vi "Test HighFrequency Client Connection.vi"() -> ()   [LabVIEW 2013]
uses:
  <vilib>/LabVIEW Open Source Project/MQTT Control Packets/Control Packets/CONNACK/Connect Return Code -- enum.ctl
  Server/Server class/Server.lvclass/Server.ctl
  Client/Client Class/Client.lvclass/Client.ctl
  <vilib>/LabVIEW Open Source Project/MQTT Control Packets/Control Packets/PUBLISH/PUBLISH.lvclass
  Server/Server class/Server.lvclass
  MQTT_Base/Base Class/MQTT_Base.lvclass
  Client/Client Class/Client.lvclass
  MQTT_TCP/Connection/TCPConnection.lvclass
  <vilib>/LabVIEW Open Source Project/MQTT Control Packets/Control Packets/CONNACK/CONNACK.lvclass
panel:
  out "NO RESPONSE":bool
  out "timed out?":bool
  out "Stop":dbl format="%.06f"
  out "Connect":dbl format="%.06f"
  out "Start":dbl format="%.06f"
  out "STOPPING":bool
  out "Waveform Chart":T1(graph)
  out "Loop period (s)":dbl format="%.06f"
  out "client Outgoing ID Request":i32
  out "Process Response":i32
  out "Process Incoming ID Request":i32
  out "Process Status":T2=enum."Server Unavailable"
  out "error server":errorcluster
  out "Client Status":T2=enum."Server Unavailable"
  out "error client process":errorcluster
  out "NbConnections":u32
  out "error client consumer":errorcluster
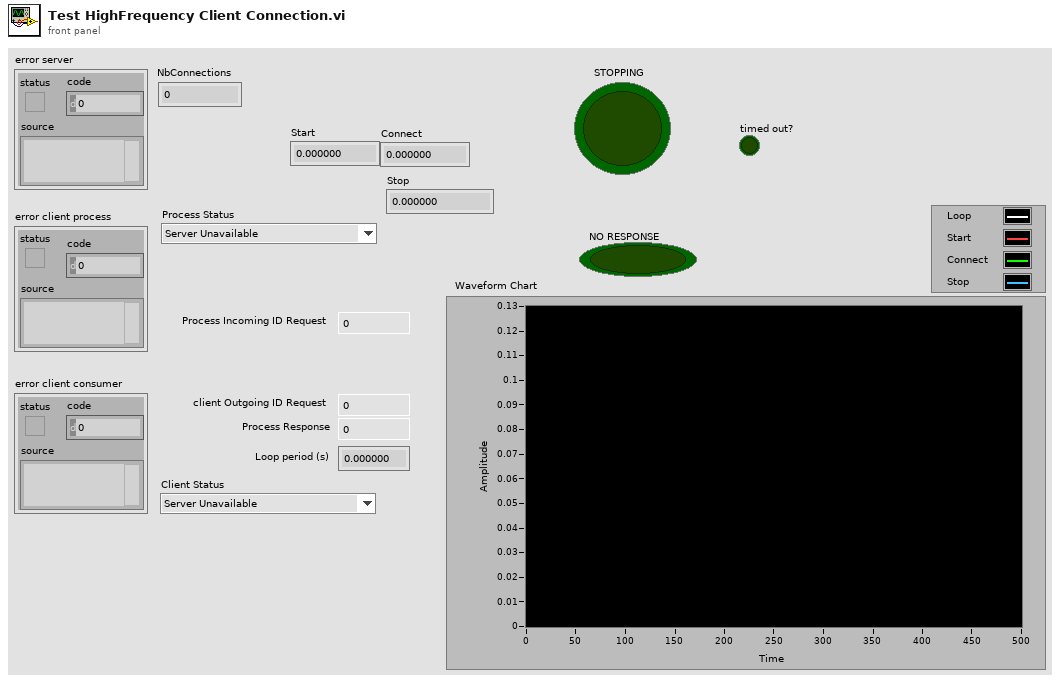
[diagram p1: front panel]
types:
  T1 = cluster{dbl, "elapsed (s)":dbl, "elapsed (s)":dbl, "elapsed (s)":dbl}
  T2 = typedef "MQTT_Control_Packets.lvlib/CONNACK.lvclass/Connect Return Code -- enum.ctl" = enum16{"Connection accepted", "Unacceptable protocol version", "Identifier Rejected", "Server Unavailable", "Bad Username or Password", "Not Authorized"}
  T3 = cluster{dbl, "elapsed (s)":dbl, "elapsed (s)":dbl, "elapsed (s)":dbl}[]
  T4 = typedef "MQTT Server.lvlib/Server.lvclass/Public Events -- cluster.ctl" = cluster{"NbConnections":refnum<user-event>}
  T5 = typedef "MQTT Client.lvlib/Client.lvclass/Public Events -- cluster.ctl" = cluster{"Connection Status":refnum<user-event>, "Connected":refnum<user-event>, "Application Message":refnum<user-event>}
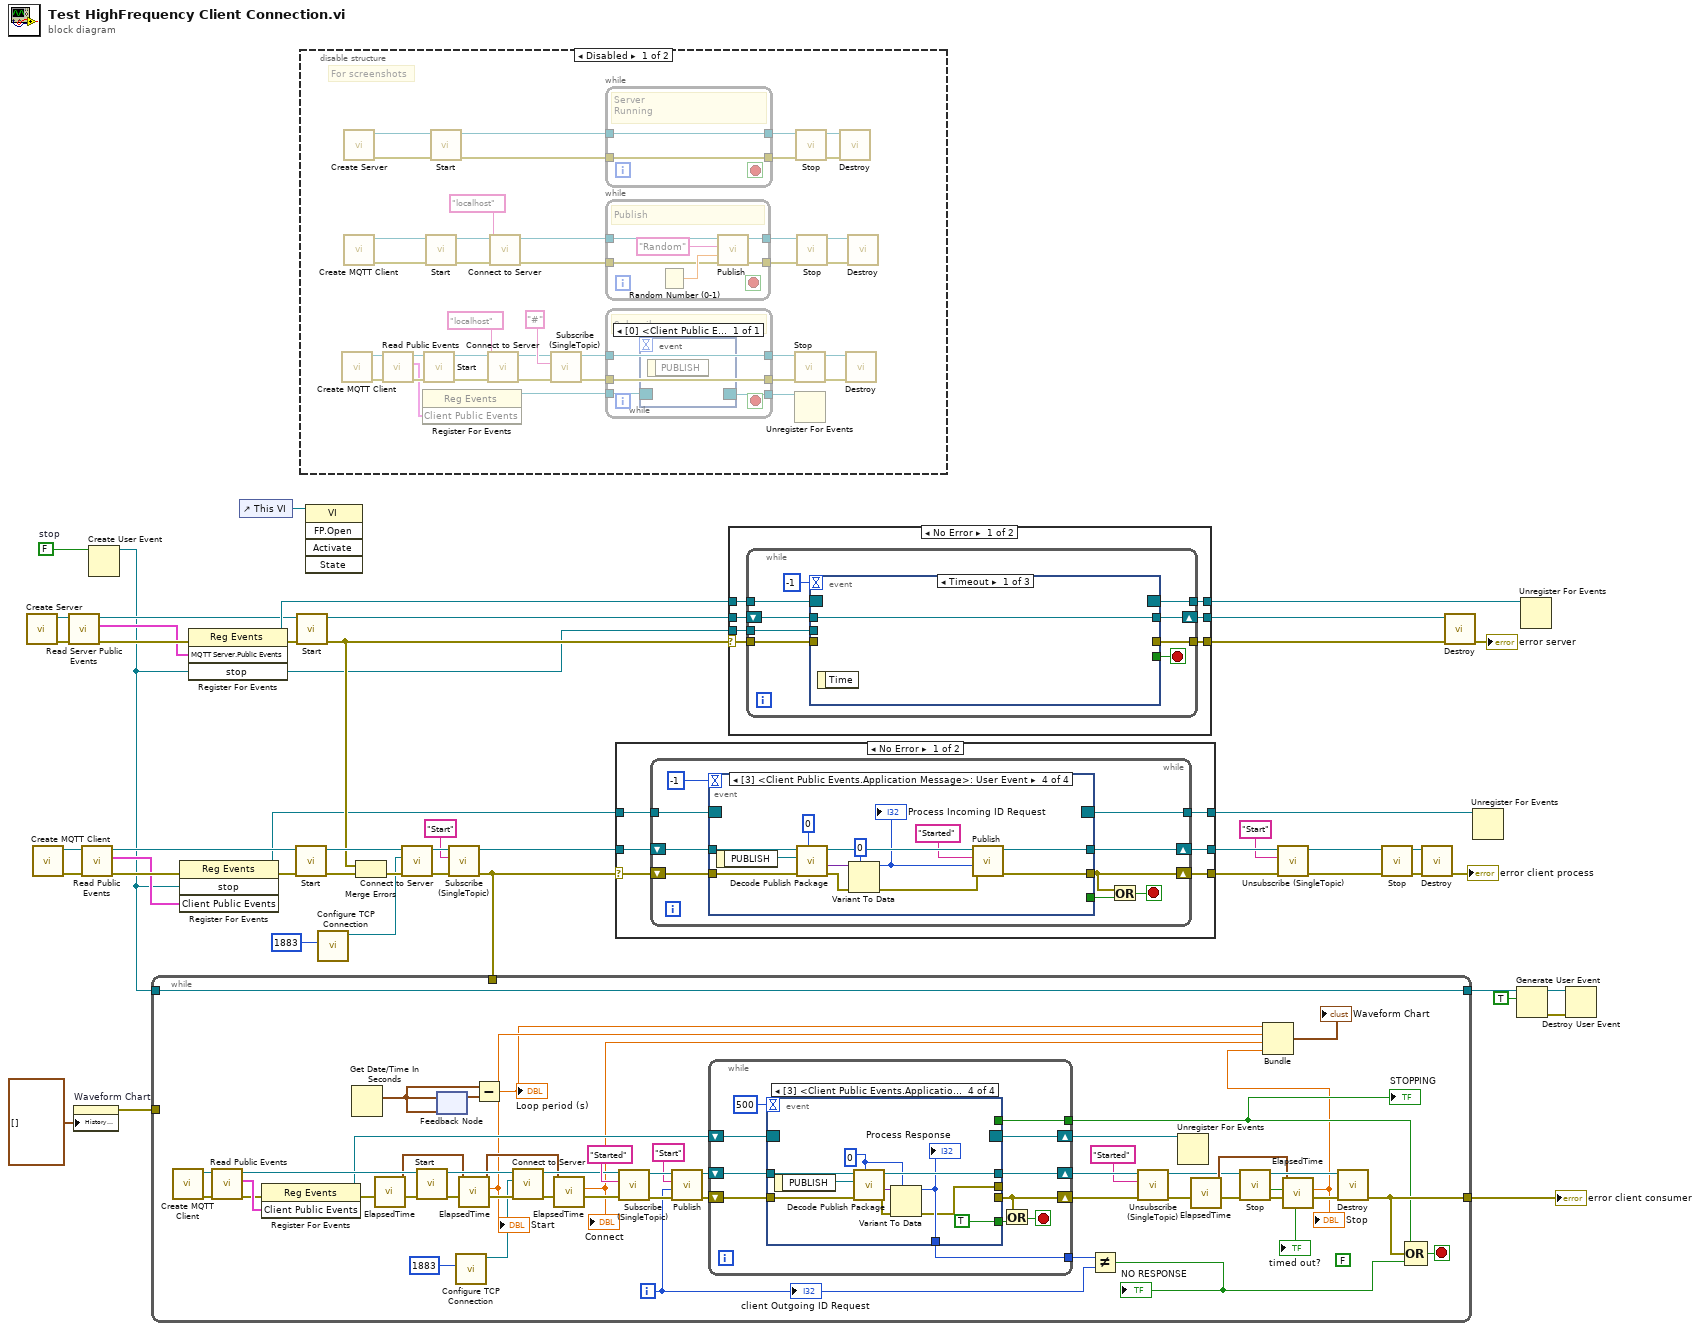
[diagram p0: block diagram]
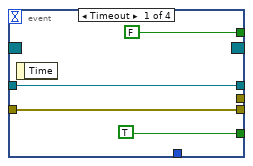
[diagram p2: hidden frame]
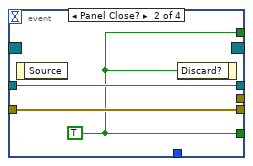
[diagram p3: hidden frame]
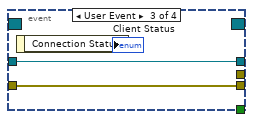
[diagram p4: hidden frame]
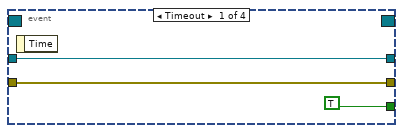
[diagram p5: hidden frame]
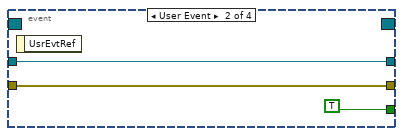
[diagram p6: hidden frame]
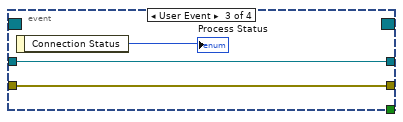
[diagram p7: hidden frame]
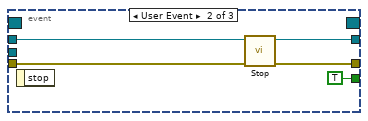
[diagram p10: hidden frame]
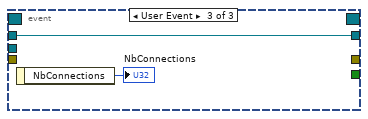
[diagram p11: hidden frame]
diagram:
  w32 = FALSE  # stop
  n1 = call "Create Server.vi"() -> ("error out"=w47:errorcluster, "Server"=w48:refnum<class "Server.lvclass">)  [unwired: 10 in]
  n2 = call "Create MQTT Client.vi"() -> ("error out"=w37:errorcluster, "Client out"=w36:refnum<class "Client.lvclass">)  [unwired: 10 in]
  n3 = call "Read Server Public Events.vi"("error in (no error)"=w47, "Server in"=w48) -> ("error out"=w46:errorcluster, "MQTT Server.Public Events"=w45:T4, "Server out"=w42:refnum<class "Server.lvclass">)  [unwired: 7 in]
  n4 = property on="Waveform Chart" class="WFChart (strict)"("History Data"=T3 []) -> (error out=w3:errorcluster)  [unwired: 2 in, 1 out]
  n5 = call "Read Public Events.vi"("error in (no error)"=w37, "Client in"=w36) -> ("error out"=w31:errorcluster, "Client Public Events"=w29:T5, "Client out"=w35:refnum<class "Client.lvclass">)  [unwired: 7 in]
  n6 = Create User Event(user event datatype=w32) -> (user event=w9:refnum<user-event>)  [unwired: 1 in, 1 out]
  n7 = register-events(error in=w31, w9, w29) -> (reference out=w21:refnum<event-registration>, error out=w30:errorcluster)  [unwired: 1 in]
  n8 = register-events(error in=w46, w45, w9) -> (reference out=w44:refnum<event-registration>, error out=w40:errorcluster)  [unwired: 1 in]
  n9 = control-ref of="This VI"() -> (w28:refnum<vi>)
  n10 = call "Start.vi"("error in (no error)"=w30, "MQTT_Base in"=w35) -> ("error out"=w33:errorcluster, "MQTT_Base out"=w34:refnum<class "Client.lvclass">)  [unwired: 7 in, 1 out]
  n11 = call "Start.vi"("error in (no error)"=w40, "MQTT_Base in"=w42) -> ("error out"=w26:errorcluster, "MQTT_Base out"=w41:refnum<class "Server.lvclass">)  [unwired: 7 in, 1 out]
  n12 = disable-structure shown="Disabled" {
    frame Disabled {
      # "For screenshots"
      n13 = call "Create MQTT Client.vi"() -> ("error out"=w54:errorcluster, "Client out"=w56:refnum<class "Client.lvclass">)  [unwired: 10 in]
      n14 = call "Create Server.vi"() -> ("error out"=w81:errorcluster, "Server"=w80:refnum<class "Server.lvclass">)  [unwired: 10 in]
      n15 = call "Create MQTT Client.vi"() -> ("error out"=w78:errorcluster, "Client out"=w79:refnum<class "Client.lvclass">)  [unwired: 10 in]
      n16 = call "Read Public Events.vi"("error in (no error)"=w54, "Client in"=w56) -> ("error out"=w53:errorcluster, "Client Public Events"=w52:T5, "Client out"=w55:refnum<class "Client.lvclass">)  [unwired: 7 in]
      n17 = register-events(w52) -> (reference out=w51:refnum<event-registration>)  [unwired: 2 in, 1 out]
      n18 = call "Start.vi"("error in (no error)"=w53, "MQTT_Base in"=w55) -> ("error out"=w71:errorcluster, "MQTT_Base out"=w72:refnum<class "Client.lvclass">)  [unwired: 7 in, 1 out]
      n19 = call "Start.vi"("error in (no error)"=w78, "MQTT_Base in"=w79) -> ("error out"=w85:errorcluster, "MQTT_Base out"=w84:refnum<class "Client.lvclass">)  [unwired: 7 in, 1 out]
      n20 = call "Start.vi"("error in (no error)"=w81, "MQTT_Base in"=w80) -> ("error out"=w63:errorcluster, "MQTT_Base out"=w65:refnum<class "Server.lvclass">)  [unwired: 7 in, 1 out]
      n21 = call "Connect to Server.vi"("error in (no error)"=w71, "Connection"="localhost" ("Topic Filter"), "Client in"=w72) -> ("error out"=w59:errorcluster, "Client out"=w60:refnum<class "Client.lvclass">)  [unwired: 5 in, 2 out]
      n22 = call "Connect to Server.vi"("error in (no error)"=w85, "Connection"="localhost" ("Topic Filter"), "Client in"=w84) -> ("error out"=w67:errorcluster, "Client out"=w70:refnum<class "Client.lvclass">)  [unwired: 5 in, 2 out]
      n23 = call "Subscribe (SingleTopic).vi"("error in (no error)"=w59, "Topic Filter"="#", "MQTT_Base in"=w60) -> ("error out"=w57:errorcluster, "MQTT_Base out"=w58:refnum<class "Client.lvclass">)  [unwired: 7 in]
      n24 = while {
        tunnel: [w99] -> w66
        tunnel: w65 -> [w99]
        tunnel: w63 -> [w98]
        tunnel: [w98] -> w64
        stop <- _ stop-if-true
        # "Server\nRunning"
      }
      n25 = while {
        tunnel: w70 -> [w95]
        tunnel: [w94] -> w69
        tunnel: [w93] -> w68
        tunnel: w67 -> [w92]
        stop <- _ stop-if-true
        # "Publish"
        n26 = Random Number (0-1)() -> (number: 0 to 1=w97:dbl)
        n27 = call "Publish.vi"("error in (no error)"=w92, "Payload"=w97, "Topic Name (empty: Payload name)"="Random", "Client in"=w95) -> ("error out"=w93:errorcluster, "Client out"=w94:refnum<class "Client.lvclass">)  [unwired: 5 in, 1 out]
      }
      n28 = while {
        tunnel: [w91] -> w61
        tunnel: w58 -> [w91]
        tunnel: w57 -> [w90]
        tunnel: [w90] -> w62
        tunnel: w51 -> [w89]
        tunnel: [w88] -> w50
        stop <- _ stop-if-true
        # "Subscribe"
        n29 = event shown="[0] <Client Public Events.Application Message>: User Event" {
          selector: w89 -> [_]
          dyn-events: [_] -> w88
          timeout: _ -> [_]
          event User Event {
            n30 = event-data() -> ()  [unwired: 1 in, 1 out]
          }
        }
      }
      n31 = call "Stop.vi"("error in (no error)"=w62, "MQTT_Base in"=w61) -> ("error out"=w74:errorcluster, "MQTT_Base out"=w75:refnum<class "Client.lvclass">)  [unwired: 7 in, 1 out]
      n32 = Unregister For Events(event registration refnum=w50) -> ()  [unwired: 1 in, 1 out]
      n33 = call "Stop.vi"("error in (no error)"=w64, "MQTT_Base in"=w66) -> ("error out"=w87:errorcluster, "MQTT_Base out"=w86:refnum<class "Server.lvclass">)  [unwired: 7 in, 1 out]
      n34 = call "Stop.vi"("error in (no error)"=w68, "MQTT_Base in"=w69) -> ("error out"=w83:errorcluster, "MQTT_Base out"=w82:refnum<class "Client.lvclass">)  [unwired: 7 in, 1 out]
      n35 = call "Destroy.vi"("error in (no error)"=w87, "MQTT_Base in"=w86) -> ()  [unwired: 8 in, 2 out]
      n36 = call "Destroy.vi"("error in (no error)"=w74, "MQTT_Base in"=w75) -> ()  [unwired: 8 in, 2 out]
      n37 = call "Destroy.vi"("error in (no error)"=w83, "MQTT_Base in"=w82) -> ()  [unwired: 8 in, 2 out]
    }
    frame Enabled {
    }
  }
  n38 = invoke class="VI" method="FP.Open"(reference=w28) -> ()  [unwired: 4 in, 5 out]
  n39 = call "Configure TCP Connection.vi"("remote port (80)"=u16 1883) -> ("TCPConnection"=w1:refnum<class "TCPConnection.lvclass">)  [unwired: 9 in, 1 out]
  n40 = Merge Errors(w26, w33) -> (w38:errorcluster)
  n41 = call "Connect to Server.vi"("error in (no error)"=w38, "Connection"=w1, "Client in"=w34) -> ("error out"=w24:errorcluster, "Client out"=w25:refnum<class "Client.lvclass">)  [unwired: 5 in, 2 out]
  n42 = call "Subscribe (SingleTopic).vi"("error in (no error)"=w24, "Topic Filter"="Start", "MQTT_Base in"=w25) -> ("error out"=w10:errorcluster, "MQTT_Base out"=w22:refnum<class "Client.lvclass">)  [unwired: 7 in]
  n43 = while {
    tunnel: [w131] -> w11
    tunnel: w10 -> [_]
    tunnel: [w129] -> w8
    tunnel: w9 -> [w129]
    tunnel: w3 -> [_]
    i -> [w130]
    stop <- w132 stop-if-true
    (unwired) FALSE
    n44 = call "Create MQTT Client.vi"() -> ("error out"=w148:errorcluster, "Client out"=w149:refnum<class "Client.lvclass">)  [unwired: 10 in]
    n45 = call "Read Public Events.vi"("error in (no error)"=w148, "Client in"=w149) -> ("error out"=w143:errorcluster, "Client Public Events"=w144:T5, "Client out"=w147:refnum<class "Client.lvclass">)  [unwired: 7 in]
    n46 = register-events(error in=w143, w144) -> (reference out=w142:refnum<event-registration>, error out=w125:errorcluster)  [unwired: 1 in]
    n47 = Get Date/Time In Seconds() -> (seconds since 1Jan1904=w127:timestamp)
    n48 = call "ElapsedTime.vi"("error in"=w125) -> ("error out"=w124:errorcluster, "current time"=w121:timestamp)  [unwired: 8 in, 1 out]
    n49 = call "Start.vi"("error in (no error)"=w124, "MQTT_Base in"=w147) -> ("error out"=w122:errorcluster, "MQTT_Base out"=w146:refnum<class "Client.lvclass">)  [unwired: 7 in, 1 out]
    n50 = feedback-in #1(w127) -> ()
    n51 = feedback #1(w127) -> (w128:timestamp)
    n52 = call "Configure TCP Connection.vi"("remote port (80)"=u16 1883) -> ("TCPConnection"=w100:refnum<class "TCPConnection.lvclass">)  [unwired: 9 in, 1 out]
    n53 = call "ElapsedTime.vi"("error in"=w122, "compare time"=w121) -> ("error out"=w123:errorcluster, "elapsed (s)"=w113:dbl, "current time"=w118:timestamp)  [unwired: 7 in]
    "Start" <- w113
    n54 = Subtract(x=w127, y=w128) -> (x-y=w110:dbl)
    "Loop period (s)" <- w110
    n55 = call "Connect to Server.vi"("error in (no error)"=w123, "Connection"=w100, "Client in"=w146) -> ("error out"=w120:errorcluster, "Client out"=w139:refnum<class "Client.lvclass">)  [unwired: 5 in, 2 out]
    n56 = call "ElapsedTime.vi"("error in"=w120, "compare time"=w118) -> ("error out"=w119:errorcluster, "elapsed (s)"=w112:dbl)  [unwired: 7 in, 1 out]
    "Connect" <- w112
    n57 = call "Subscribe (SingleTopic).vi"("error in (no error)"=w119, "Topic Filter"="Started", "MQTT_Base in"=w139) -> ("error out"=w138:errorcluster, "MQTT_Base out"=w137:refnum<class "Client.lvclass">)  [unwired: 7 in]
    n58 = call "Publish.vi"("error in (no error)"=w138, "Payload"=w130, "Topic Name (empty: Payload name)"="Start" ("Topic Filter"), "Client in"=w137) -> ("error out"=w135:errorcluster, "Client out"=w136:refnum<class "Client.lvclass">)  [unwired: 5 in, 1 out]
    n59 = while {
      shift-right: [w158] -> w106
      shift-left: w136 -> [w154]
      shift-right: [w159] -> w141
      shift-left: w142 -> [w160]
      shift-right: [w157] -> w104
      shift-left: w135 -> [w153]
      tunnel: [w151] -> w133
      tunnel: [w150] -> w126
      stop <- w152 stop-if-true
      n60 = event shown="[3] <Client Public Events.Application Message>: User Event" {
        selector: w160 -> [_ _ _ _]
        dyn-events: [_ _ _ _] -> w159
        timeout: 500 -> [_ _ _ _]
        tunnel: w154 -> [w163 w167 w169 w179]
        tunnel: [w163 w167 w169 w177] -> w158
        tunnel: [w162 w166 w168 _] -> w157
        tunnel: w153 -> [w162 w166 w168 w176]
        tunnel: [TRUE w165 _ TRUE] -> w156
        tunnel: [_ _ _ w172] -> w151
        tunnel: [FALSE w165 _ _] -> w150
        tunnel: [_ _ _ w171] -> _
        event Timeout {
          n61 = event-data() -> ()  [unwired: 1 in, 1 out]
        }
        event Panel Close? {
          w165 = TRUE
          n62 = event-data() -> ()  [unwired: 1 in, 1 out]
          n63 = event-data("Discard?"=w165) -> ()  [unwired: 1 in, 1 out]
        }
        event User Event {
          n64 = event-data() -> ("Connection Status"=→"Client Status":T2)  [unwired: 1 in]
        }
        event User Event {
          w175 = 0
          n65 = event-data() -> ("PUBLISH"=w180:refnum<class "PUBLISH.lvclass">)  [unwired: 1 in]
          n66 = call "Decode Publish Package.vi"("Type"=w175, "error in (no error)"=w176, "PUBLISH in"=w180, "MQTT_Base in"=w179) -> ("error out"=w174:errorcluster, "Payload"=w178:variant, "MQTT_Base out"=w177:refnum<class "Client.lvclass">)  [unwired: 4 in, 1 out]
          n67 = Variant To Data(error in=w174, type=w175, Variant=w178) -> (data=w172:i32, error out=w171:errorcluster)
          "Process Response" <- w172
        }
      }
      n68 = Or(x=w157, y=w156) -> (x .or. y?=w152:bool)
    }
    "STOPPING" <- w126
    n69 = Not Equal?(x=w133, y=w130) -> (x != y?=w107:bool)
    "NO RESPONSE" <- w107
    n70 = call "Unsubscribe (SingleTopic).vi"("error in (no error)"=w104, "Topic Filter"="Started", "MQTT_Base in"=w106) -> ("error out"=w103:errorcluster, "MQTT_Base out"=w105:refnum<class "Client.lvclass">)  [unwired: 7 in]
    n71 = Unregister For Events(event registration refnum=w141) -> ()  [unwired: 1 in, 1 out]
    n72 = call "ElapsedTime.vi"("error in"=w103) -> ("error out"=w117:errorcluster, "current time"=w114:timestamp)  [unwired: 8 in, 1 out]
    n73 = call "Stop.vi"("error in (no error)"=w117, "MQTT_Base in"=w105) -> ("error out"=w115:errorcluster, "timed out?"=→"timed out?":bool, "MQTT_Base out"=w145:refnum<class "Client.lvclass">)  [unwired: 7 in]
    n74 = call "ElapsedTime.vi"("error in"=w115, "compare time"=w114) -> ("error out"=w116:errorcluster, "elapsed (s)"=w111:dbl)  [unwired: 7 in, 1 out]
    "Stop" <- w111
    n75 = Bundle(w110, "elapsed (s)"=w113, "elapsed (s)"=w112, "elapsed (s)"=w111) -> (→"Waveform Chart":T1)  [unwired: 1 in]
    n76 = call "Destroy.vi"("error in (no error)"=w116, "MQTT_Base in"=w145) -> ("error out"=w131:errorcluster)  [unwired: 8 in, 1 out]
    n77 = Compound Arithmetic op=OR(w126, w131, w107) -> (w132:bool)
    "client Outgoing ID Request" <- w130
  }
  "error client consumer" <- w11
  n78 = case shown="No Error" w10 {
    selector: w10 -> [w181 w218]
    tunnel: w21 -> [w186 w220]
    tunnel: [w185 w220] -> w17
    tunnel: w22 -> [w184 w219]
    tunnel: [w183 w219] -> w15
    tunnel: [w182 w218] -> w13
    frame No Error {
      n79 = while {
        tunnel: w186 -> [w195]
        tunnel: [w194] -> w185
        shift-right: [w192] -> w183
        shift-left: w184 -> [w193]
        shift-right: [w189] -> w182
        shift-left: w181 -> [w191]
        stop <- w190 stop-if-true
        n80 = event shown="[3] <Client Public Events.Application Message>: User Event" {
          selector: w195 -> [_ _ _ _]
          dyn-events: [_ _ _ _] -> w194
          timeout: -1 -> [_ _ _ _]
          tunnel: w193 -> [w197 w200 w203 w216]
          tunnel: [w197 w200 w203 w209] -> w192
          tunnel: [w196 w199 w202 w205] -> w189
          tunnel: w191 -> [w196 w199 w202 w213]
          tunnel: [TRUE TRUE _ _] -> w188
          event Timeout {
            n81 = event-data() -> ()  [unwired: 1 in, 1 out]
          }
          event User Event {
            n82 = event-data() -> ()  [unwired: 1 in, 1 out]
          }
          event User Event {
            n83 = event-data() -> ("Connection Status"=→"Process Status":T2)  [unwired: 1 in]
          }
          event User Event {
            n84 = event-data() -> ("PUBLISH"=w217:refnum<class "PUBLISH.lvclass">)  [unwired: 1 in]
            n85 = call "Decode Publish Package.vi"("Type"=0, "error in (no error)"=w213, "PUBLISH in"=w217, "MQTT_Base in"=w216) -> ("error out"=w212:errorcluster, "Payload"=w215:variant, "MQTT_Base out"=w210:refnum<class "Client.lvclass">)  [unwired: 4 in, 1 out]
            n86 = Variant To Data(error in=w212, type=0, Variant=w215) -> (data=w207:i32, error out=w206:errorcluster)
            "Process Incoming ID Request" <- w207
            n87 = call "Publish.vi"("error in (no error)"=w206, "Payload"=w207, "Topic Name (empty: Payload name)"="Started" ("Topic Filter"), "Client in"=w210) -> ("error out"=w205:errorcluster, "Client out"=w209:refnum<class "Client.lvclass">)  [unwired: 5 in, 1 out]
          }
        }
        n88 = Or(x=w189, y=w188) -> (x .or. y?=w190:bool)
      }
    }
    frame Error {
    }
  }
  n89 = case shown="No Error" w26 {
    selector: w26 -> [w221 w245]
    tunnel: w41 -> [w227 w247]
    tunnel: [w226 w247] -> w49
    tunnel: w44 -> [w225 w246]
    tunnel: [w224 w246] -> w43
    tunnel: [w223 w245] -> w39
    tunnel: w9 -> [w222 _]
    frame No Error {
      n90 = while {
        shift-right: [w233] -> w226
        shift-left: w227 -> [w235]
        tunnel: w225 -> [w232]
        tunnel: [w231] -> w224
        tunnel: [w230] -> w223
        tunnel: w222 -> [w229]
        tunnel: w221 -> [w228]
        stop <- w234 stop-if-true
        n91 = event shown="[0] Timeout" {
          selector: w232 -> [_ _ _]
          dyn-events: [_ _ _] -> w231
          timeout: -1 -> [_ _ _]
          tunnel: w235 -> [w237 w242 w244]
          tunnel: [_ TRUE ("Discard?") _] -> w234
          tunnel: [w237 w241 w244] -> w233
          tunnel: [_ w240 _] -> w230
          tunnel: w229 -> [_ _ _]
          tunnel: w228 -> [_ w238 _]
          event Timeout {
            n92 = event-data() -> ()  [unwired: 1 in, 1 out]
          }
          event User Event {
            n93 = event-data() -> ()  [unwired: 1 in, 1 out]
            n94 = call "Stop.vi"("error in (no error)"=w238, "MQTT_Base in"=w242) -> ("error out"=w240:errorcluster, "MQTT_Base out"=w241:refnum<class "Server.lvclass">)  [unwired: 7 in, 1 out]
          }
          event User Event {
            n95 = event-data() -> ("NbConnections"=→"NbConnections":u32)  [unwired: 1 in]
          }
        }
      }
    }
    frame Error {
    }
  }
  n96 = call "Unsubscribe (SingleTopic).vi"("error in (no error)"=w13, "Topic Filter"="Start", "MQTT_Base in"=w15) -> ("error out"=w14:errorcluster, "MQTT_Base out"=w16:refnum<class "Client.lvclass">)  [unwired: 7 in]
  n97 = call "Stop.vi"("error in (no error)"=w14, "MQTT_Base in"=w16) -> ("error out"=w19:errorcluster, "MQTT_Base out"=w20:refnum<class "Client.lvclass">)  [unwired: 7 in, 1 out]
  n98 = call "Destroy.vi"("error in (no error)"=w19, "MQTT_Base in"=w20) -> ("error out"=→"error client process":errorcluster)  [unwired: 8 in, 1 out]
  n99 = call "Destroy.vi"("error in (no error)"=w39, "MQTT_Base in"=w49) -> ("error out"=→"error server":errorcluster)  [unwired: 8 in, 1 out]
  n100 = Unregister For Events(event registration refnum=w17) -> ()  [unwired: 1 in, 1 out]
  n101 = Generate User Event(user event=w8, event data cluster=TRUE ("event data")) -> (user event out=w6:refnum<user-event>, error out=w7:errorcluster)  [unwired: 2 in]
  n102 = Unregister For Events(event registration refnum=w43) -> ()  [unwired: 1 in, 1 out]
  n103 = Destroy User Event(user event=w6, error in=w7) -> ()  [unwired: 1 out]
